vi "2P_AdapUprite_Linlin.vi"() -> ()   [LabVIEW 2015] (continued)
                                }
                                }
                                }
                                n1665 = Build Array(w4642) -> (w4641:T20)
                                }
                                }
                                }
                                frame #9 {
                                n1666 = Build Array(w4671, w4670) -> (w4673:bool[])
                                n1667 = Boolean Array To Number(Boolean array=w4673) -> (number=w4672:u32)
                                n1668 = case shown="0" w4672 {
                                tunnel: w4669 -> [_ w4725 _ w4729]
                                tunnel: [_ w4720 _ w4726] -> w4668
                                frame 1 {
                                n1669 = call "2pparameters.vi"("command"="get") -> ("params out"=w4680:T12)  [unwired: 1 in]
                                n1670 = Unbundle By Name(w4680) -> ("wavdet"=w4681:bool, "Pel"=w4683:sgl, "refwfsize"=w4684:dbl, "Pel"=w4682:sgl)
                                n1671 = call "waveformsDObuffer.vi"("command"="get") -> ("DO wf out"=w4676:digitalwaveform[])  [unwired: 1 in]
                                n1672 = case shown="True" w4681 {
                                tunnel: [w4688 w4701] -> w4678
                                tunnel: w4682 -> [w4697 w4716]
                                tunnel: w4683 -> [w4687 w4707]
                                tunnel: w4684 -> [_ w4713]
                                frame False {
                                w4691 = u16 0 items=["unsigned binary", "offset binary", "2's complement"] ("data format (offset binary)")
                                n1673 = Initialize Array(sgl 0.0, w4687) -> (w4694:sgl[])
                                n1674 = Replace Array Subset(array=w4694, new element=sgl 1.0, index=0) -> (w4692:sgl[])
                                n1675 = Reciprocal(x=w4697) -> (1/x=w4698:sgl)
                                n1676 = Bundle By Name("Y"=w4692, "dt"=w4698) -> (w4689:waveform(sgl))  [unwired: 1 in]
                                n1677 = call-poly <vilib>:"Analog to Digital.vi"("data format (offset binary)"=w4691, "compress digital (T)"=TRUE, "full-scale range (pk-pk)"=1.0, "resolution (16 bit)"=1, "analog waveform"=w4689) -> ("digital waveform"=w4688:digitalwaveform)  [unwired: 3 in, 3 out]
                                }
                                frame True {
                                w4704 = u16 0 items=["unsigned binary", "offset binary", "2's complement"] ("data format (offset binary)")
                                n1678 = To Double Precision Float(number=w4707) -> (double precision float=w4714:dbl)
                                n1679 = Initialize Array(sgl 0.0, w4707) -> (w4709:sgl[])
                                n1680 = Divide(x=w4713, y=w4714) -> (x/y=w4711:dbl)
                                n1681 = Round Toward +Infinity(x=w4711) -> (ceil(x): smallest int >= x=w4712:dbl)
                                n1682 = Replace Array Subset(array=w4709, new element=sgl 1.0, index=0) -> (w4706:sgl[])
                                n1683 = for {
                                N: w4712 -> [_]
                                tunnel: w4706 -> [w4718]
                                tunnel: [w4718] -> w4715 mode=concatenating
                                }
                                n1684 = Reciprocal(x=w4716) -> (1/x=w4717:sgl)
                                n1685 = Bundle By Name("Y"=w4715, "dt"=w4717) -> (w4702:waveform(sgl))  [unwired: 1 in]
                                n1686 = call-poly <vilib>:"Analog to Digital.vi"("data format (offset binary)"=w4704, "compress digital (T)"=TRUE, "full-scale range (pk-pk)"=1.0, "resolution (16 bit)"=1, "analog waveform"=w4702) -> ("digital waveform"=w4701:digitalwaveform)  [unwired: 3 in, 3 out]
                                }
                                }
                                n1687 = Build Array (concatenate)(w4676, w4678) -> (w4674:digitalwaveform[])
                                n1688 = call "waveformsDObuffer.vi"("DO wf in"=w4674, "command"="set") -> ()  [unwired: 1 out]
                                }
                                frame 2 {
                                n1689 = call "waveformsDObuffer.vi"("command"="get") -> ("DO wf out"=w4722:digitalwaveform[])  [unwired: 1 in]
                                n1690 = Delete From Array(array=w4722, length=1, index=w4725) -> (deleted portion=w4720:digitalwaveform[], array with subset deleted=w4719:digitalwaveform[])
                                n1691 = call "waveformsDObuffer.vi"("DO wf in"=w4719, "command"="set") -> ()  [unwired: 1 out]
                                }
                                frame 3, Default {
                                }
                                frame 0 {
                                n1692 = local read "Measurement"() -> (w4728:T4)
                                n1693 = To Unsigned Long Integer(number=w4728) -> (unsigned 32bit integer=w4727:u32)
                                n1694 = case shown="5..7" w4727 {
                                tunnel: w4729 -> [_ w4732]
                                tunnel: [_ w4731] -> w4726
                                frame 0..4, Default {
                                }
                                frame 5..7 {
                                n1695 = call "2pparameters.vi"("command"="get") -> ("params out"=w4739:T12)  [unwired: 1 in]
                                n1696 = Unbundle By Name(w4739) -> ("wavdet"=w4740:bool, "Pel"=w4742:sgl, "refwfsize"=w4743:dbl, "srateAODO"=w4741:sgl)
                                n1697 = call "waveformsDObuffer.vi"("command"="get") -> ("DO wf out"=w4733:digitalwaveform[])  [unwired: 1 in]
                                n1698 = Index Array(array=w4733, index=w4732) -> (element=w4734:digitalwaveform)
                                n1699 = case shown="True" w4740 {
                                tunnel: [w4747 w4760] -> w4737
                                tunnel: w4741 -> [w4756 w4775]
                                tunnel: w4742 -> [w4746 w4766]
                                tunnel: w4743 -> [_ w4772]
                                frame False {
                                w4750 = u16 0 items=["unsigned binary", "offset binary", "2's complement"] ("data format (offset binary)")
                                n1700 = Initialize Array(sgl 0.0, w4746) -> (w4753:sgl[])
                                n1701 = Replace Array Subset(array=w4753, new element=sgl 1.0, index=0) -> (w4751:sgl[])
                                n1702 = Reciprocal(x=w4756) -> (1/x=w4757:sgl)
                                n1703 = Bundle By Name("Y"=w4751, "dt"=w4757) -> (w4748:waveform(sgl))  [unwired: 1 in]
                                n1704 = call-poly <vilib>:"Analog to Digital.vi"("data format (offset binary)"=w4750, "compress digital (T)"=TRUE, "full-scale range (pk-pk)"=1.0, "resolution (16 bit)"=1, "analog waveform"=w4748) -> ("digital waveform"=w4747:digitalwaveform)  [unwired: 3 in, 3 out]
                                }
                                frame True {
                                w4763 = u16 0 items=["unsigned binary", "offset binary", "2's complement"] ("data format (offset binary)")
                                n1705 = To Double Precision Float(number=w4766) -> (double precision float=w4773:dbl)
                                n1706 = Initialize Array(sgl 0.0, w4766) -> (w4768:sgl[])
                                n1707 = Divide(x=w4772, y=w4773) -> (x/y=w4770:dbl)
                                n1708 = Round Toward +Infinity(x=w4770) -> (ceil(x): smallest int >= x=w4771:dbl)
                                n1709 = Replace Array Subset(array=w4768, new element=sgl 1.0, index=0) -> (w4765:sgl[])
                                n1710 = for {
                                N: w4771 -> [_]
                                tunnel: w4765 -> [w4777]
                                tunnel: [w4777] -> w4774 mode=concatenating
                                }
                                n1711 = Reciprocal(x=w4775) -> (1/x=w4776:sgl)
                                n1712 = Bundle By Name("Y"=w4774, "dt"=w4776) -> (w4761:waveform(sgl))  [unwired: 1 in]
                                n1713 = call-poly <vilib>:"Analog to Digital.vi"("data format (offset binary)"=w4763, "compress digital (T)"=TRUE, "full-scale range (pk-pk)"=1.0, "resolution (16 bit)"=1, "analog waveform"=w4761) -> ("digital waveform"=w4760:digitalwaveform)  [unwired: 3 in, 3 out]
                                }
                                }
                                n1714 = Build Array(w4734) -> (w4731:digitalwaveform[])
                                n1715 = Replace Array Subset(array=w4733, new element=w4737, index=w4732) -> (w4730:digitalwaveform[])
                                n1716 = call "waveformsDObuffer.vi"("DO wf in"=w4730, "command"="set") -> ()  [unwired: 1 out]
                                }
                                }
                                }
                                }
                                }
                                frame #10 {
                                # "Source of crashing?"
                                n1717 = local read "Meastab"() -> (w4791:enum32{"X-Y Image", "Linescan", "Timetrace"})
                                n1718 = property on="refwf" class="Ring (strict)"() -> ("RingText.Text"=w4788:string)  [unwired: 2 in, 2 out]
                                n1719 = case shown="\"Timetrace\"" w4791 {
                                tunnel: [w4793 w4794] -> w4792
                                frame "X-Y Image", Default {
                                n1720 = local read "Sampling rate"() -> (w4793:dbl)
                                }
                                frame "Timetrace" {
                                n1721 = local read "srateAODOtt"() -> (w4794:dbl)
                                }
                                }
                                n1722 = call "waveformsAObuffer.vi"("command"="get") -> ("AO wf out"=w4781:waveform(dbl)[])  [unwired: 1 in]
                                n1723 = local read "wavdet"() -> (w4789:bool)
                                n1724 = call "waveformsDObuffer.vi"("command"="get") -> ("DO wf out"=w4785:digitalwaveform[])  [unwired: 1 in]
                                n1725 = call "correctwaveformsizetemp.vi"("new sampling frequency (Hz)"=w4792, "start"=TRUE, "reference waveforms to"=w4788, "Analog waveforms in"=w4781, "stop"=FALSE, "Digital waveforms in"=w4785) -> ("analog wf out"=w4787:waveform(dbl)[], "Digital wf out"=w4780:digitalwaveform[], "measpoints"=w4790:i32)
                                n1726 = call "waveformsDObuffer.vi"("DO wf in"=w4780, "command"="set") -> ()  [unwired: 1 out]
                                n1727 = call "waveformsAObuffer.vi"("AO wf in"=w4787, "command"="set") -> ()  [unwired: 1 out]
                                n1728 = case shown="True" w4789 {
                                tunnel: w4790 -> [_ w4797]
                                tunnel: w4780 -> [_ w4795]
                                frame False {
                                }
                                frame True {
                                n1729 = local write "# of frames"(w4797) -> ()
                                n1730 = call "GetNumCamFramesv2.vi"("Digital Waveform Graph"=w4795) -> ("Numeric"=w4796:i32)  [unwired: 10 in]
                                n1731 = local write "Total Camera Frames"(w4796) -> ()
                                }
                                }
                                }
                                }
                              }
                              frame #7 {
                                # "Disabled for conversion to 64 bit"
                                # "lifetime related stuff"
                                n1732 = disable-structure shown="Disabled" {
                                frame Disabled {
                                n1733 = local read "Measurement"() -> (w4799:T4)
                                n1734 = case shown="\"Lifetime (scan)\"" w4799 {
                                frame "X-Y-t movie", Default {
                                }
                                frame "Lifetime (scan)" {
                                # "total acquisition time"
                                n1735 = call "2pparameters.vi"("command"="get") -> ("params out"=w4807:T12)  [unwired: 1 in]
                                n1736 = Unbundle By Name(w4807) -> ("measpoints"=w4801:i32, "srateAODO"=w4822:sgl)
                                n1737 = Divide(x=w4801, y=w4822) -> (x/y=w4800:sgl)
                                n1738 = local read "min phot"() -> (w4817:u32)
                                n1739 = local read "expected c/s"() -> (w4818:dbl)
                                n1740 = Multiply(x=w4800, y=1000.0) -> (x*y=w4810:dbl)
                                n1741 = local read "truncate"() -> (w4816:u32)
                                n1742 = To Long Integer(number=w4810) -> (32bit integer=w4819:i32)
                                n1743 = To Long Integer(number=w4818) -> (32bit integer=w4820:i32)
                                n1744 = local read "Number of Bins"() -> (w4811:u32)
                                n1745 = local read item#-1() -> (w4815)
                                n1746 = local write "Acquisition time"(w4819) -> ()
                                n1747 = local read item#-1() -> (w4813)
                                n1748 = local read item#-1() -> (w4814)
                                n1749 = local read item#-1() -> (w4812)
                                n1750 = call "lifetimeparameters.vi"("command"="get") -> ("Params out"=w4805:T22)  [unwired: 1 in]
                                n1751 = Add(x=100, y=w4819) -> (x+y=w4809:i32)
                                n1752 = Bundle By Name(cluster=w4805, "acq time"=w4809, "acq rate"=w4820, "# bins"=w4811, "Ch0 Level"=w4812, "Ch1 Level"=w4813, "Ch0 ZeroX"=w4814, "Ch1 ZeroX"=w4815, "min photons"=w4817, "truncate"=w4816) -> (w4804:T22)
                                n1753 = local write "Acquisition rate"(w4820) -> ()
                                n1754 = call "lifetimeparameters.vi"("Params in"=w4804, "command"="set") -> ()  [unwired: 1 out]
                                }
                                }
                                }
                                frame Enabled {
                                }
                                }
                                n1755 = local write "64bit disabled"(TRUE ("64bit disabled")) -> ()
                              }
                              frame #8 {
                                # "setting timeout and sample mode"
                                n1756 = call "2pparameters.vi"("command"="get") -> ("params out"=w4833:T12)  [unwired: 1 in]
                                n1757 = Unbundle By Name(w4833) -> ("refreshbuffer"=w4831:i32, "srate"=w4832:sgl)
                                n1758 = local read "wavdet"() -> (w4823:bool)
                                n1759 = To Double Precision Float(number=w4832) -> (double precision float=w4835:dbl)
                                n1760 = To Double Precision Float(number=w4831) -> (double precision float=w4826:dbl)
                                n1761 = case shown="False" w4823 {
                                tunnel: [w4840 w4841] -> w4825
                                frame False {
                                w4840 = 10123 items=["Finite Samples"=10178, "Continuous Samples"=10123, "Hardware Timed Single Point"=12522] ("sample mode")
                                }
                                frame True {
                                w4841 = 10123 items=["Finite Samples"=10178, "Continuous Samples"=10123, "Hardware Timed Single Point"=12522] ("sample mode")
                                }
                                }
                                n1762 = Divide(x=w4826, y=w4835) -> (x/y=w4839:dbl)
                                n1763 = Multiply(x=w4839, y=2.0) -> (x*y=w4836:dbl)
                                n1764 = Max & Min(x=w4836, y=10.0) -> (max(x,y)=w4827:dbl)  [unwired: 1 out]
                                n1765 = call "2pparameters.vi"("command"="get") -> ("params out"=w4830:T12)  [unwired: 1 in]
                                n1766 = Bundle By Name(cluster=w4830, "timeout"=w4827, "sample mode"=w4825) -> (w4828:T12)
                                n1767 = call "2pparameters.vi"("Params in"=w4828, "command"="set") -> ()  [unwired: 1 out]
                              }
                            }
                          }
                          frame #1 {
                            # "waveform prepped in prep AO img"
                            # "Disabled for conversion to 64 bit"
                            # "start preparing the tasks"
                            n1768 = call "prepAO_img.vi"() -> ("Terminal Name with Device Prefix"=w4843:tag)
                            n1769 = call "prepDO_img.vi"() -> ()  [unwired: 2 in]
                            n1770 = call "prepAI_img.vi"("triggersource"=w4843) -> ()  [unwired: 2 in]
                            n1771 = call "prepCI_img.vi"("ArmStart.DigEdge.Src"=w4843) -> ()  [unwired: 1 in]
                            n1772 = disable-structure shown="Disabled" {
                              frame Disabled {
                                n1773 = local read "Measurement"() -> (w4844:T4)
                                n1774 = case shown="\"Lifetime (contour)\"" w4844 {
                                frame "X-Y-t movie", Default {
                                }
                                frame "Lifetime (contour)" {
                                n1775 = stacked-sequence {
                                frame #0 {
                                n1776 = call "PH-temp.vi"("String"="clear" ("command")) -> ()  [unwired: 2 in, 2 out]
                                n1777 = call "PH-temp-raw.vi"("command"="empty") -> ()  [unwired: 1 in, 1 out]
                                }
                                frame #1 {
                                n1778 = call "calib.vi"() -> ()  [unwired: 1 in]
                                }
                                frame #2 {
                                n1779 = call "setup.vi"() -> ()  [unwired: 1 in]
                                }
                                }
                                }
                                }
                              }
                              frame Enabled {
                              }
                            }
                            n1780 = local write "64bit disabled"(TRUE ("64bit disabled")) -> ()
                          }
                          frame #2 {
                            # "prepares files for saving"
                            n1781 = local read "save\ndata"() -> (w4847:bool)
                            n1782 = case shown="True" w4847 {
                              tunnel: w4848 -> [_ w4852]
                              frame False {
                              }
                              frame True {
                                n1783 = local read "filename prefix"() -> (w4850:string)
                                n1784 = local read "data dir"() -> (w4851:path)
                                n1785 = call "preparebinaryfiles.vi"("filename prefix"=w4850, "data dir"=w4851, "timestamp"=w4852) -> ("full-filename"=w4849:string)  [unwired: 1 in]
                                n1786 = local write "full-filename"(w4849) -> ()
                              }
                            }
                            n1787 = call "preptempbuffers_tt.vi"() -> ()  [unwired: 12 in]
                          }
                          frame #3 {
                            n1788 = local read "wavdet"() -> (w4853:bool)
                            n1789 = case shown="False" w4853 {
                              frame False {
                                n1790 = disable-structure shown="Disabled" {
                                frame Disabled {
                                n1791 = call "2pparameters.vi"("command"="get") -> ("params out"=w4856:T12)  [unwired: 1 in]
                                n1792 = Unbundle By Name(w4856) -> ("autoshutter"=w4857:bool, "aAS"=w4854:u32[])
                                n1793 = case shown="True" w4857 {
                                tunnel: w4854 -> [_ w4858]
                                frame False {
                                }
                                frame True {
                                n1794 = call "shuttercontrol_multi.vi"("Autoshutter Chans"=w4858, "command"="open") -> ()  [unwired: 1 in, 1 out]
                                }
                                }
                                }
                                frame Enabled {
                                }
                                }
                              }
                              frame True {
                              }
                            }
                          }
                          frame #4 {
                            # "start trigger comes from AO, so  start everything and then start AO"
                            n1795 = flat-sequence {
                              frame #0 {
                                # "Disabled for conversion to 64 bit"
                                n1796 = disable-structure shown="Disabled" {
                                frame Disabled {
                                n1797 = local read "Measurement"() -> (w4861:T4)
                                n1798 = case shown="\"Lifetime (contour)\"" w4861 {
                                frame "X-Y-t movie", Default {
                                }
                                frame "Lifetime (contour)" {
                                n1799 = call "runLT_img.vi"() -> ()  [unwired: 1 in]
                                }
                                }
                                }
                                frame Enabled {
                                }
                                }
                                n1800 = local write "64bit disabled"(TRUE ("64bit disabled")) -> ()
                              }
                              frame #1 {
                                n1801 = call "runAI_img.vi"() -> ()  [unwired: 12 in]
                                n1802 = call "runCI.vi"() -> ()  [unwired: 12 in]
                                n1803 = call "runDO_img.vi"() -> ()  [unwired: 12 in]
                              }
                              frame #2 {
                                n1804 = call "runAO_img.vi"() -> ()  [unwired: 12 in]
                              }
                            }
                          }
                          frame #5 {
                            # "Disabled for conversion to 64 bit"
                            n1805 = while {
                              i -> [w4887]
                              stop <- w4885 stop-if-true
                              n1806 = local read "Stop"() -> (w4895:bool)
                              n1807 = local read "Exit"() -> (w4894:bool)
                              n1808 = Or(x=w4895, y=w4894) -> (x .or. y?=w4893:bool)
                              n1809 = case shown="False" w4893 {
                                frame False {
                                n1810 = stacked-sequence {
                                frame #0 {
                                n1811 = call "collectAI_tt_V2.vi"() -> ()  [unwired: 4 in]
                                n1812 = call "collectCI_tt.vi"() -> ("size(s)"=w4902:i32)  [unwired: 3 in]
                                n1813 = local write "scol"(w4902) -> ()
                                }
                                frame #1 {
                                n1814 = local read "Live"() -> (w4903:bool)
                                n1815 = case shown="True" w4903 {
                                frame False {
                                }
                                frame True {
                                n1816 = local read "graph1list"() -> (w4910:u16)
                                n1817 = local read "graph2list"() -> (w4909:u16)
                                n1818 = To Unsigned Word Integer(number=w4910) -> (unsigned 16bit integer=w4908:u16)
                                n1819 = To Unsigned Word Integer(number=w4909) -> (unsigned 16bit integer=w4907:u16)
                                n1820 = call "dattotrace.vi"("graph2list"=w4907, "Current Average"=sgl 1.0, "graph1list"=w4908) -> ("trace2array out"=w4905:sgl[], "trace1array out"=w4916:sgl[])
                                n1821 = local read "bin"() -> (w4917:dbl)
                                n1822 = script code="data=reshape(datain,[bin length(datain)./bin]);\ndataout=mean(data,1);\ndata2=reshape(datain2,[bin length(datain2)./bin]);\ndataout2=mean(data2,1);"("bin"=w4917, "datain"=w4916, "datain2"=w4905) -> ("dataout"=w4915:dbl[], "dataout2"=w4904:dbl[])  [unwired: 1 in, 1 out]
                                n1823 = Array Size(array=w4904) -> (size(s)=w4918:i32)
                                n1824 = Divide(x=w4918, y=2) -> (x/y=w4920:dbl)
                                n1825 = Round To Nearest(number=w4920) -> (nearest integer value=w4922:dbl)
                                n1826 = Array Size(array=w4915) -> (size(s)=w4927:i32)
                                n1827 = Delete From Array(array=w4904, length=w4922, index=0) -> (deleted portion=w4913:dbl[], array with subset deleted=w4914:dbl[])
                                n1828 = Divide(x=w4927, y=2) -> (x/y=w4925:dbl)
                                n1829 = Round To Nearest(number=w4925) -> (nearest integer value=w4923:dbl)
                                n1830 = Delete From Array(array=w4915, length=w4923, index=0) -> (deleted portion=w4912:dbl[], array with subset deleted=w4911:dbl[])
                                n1831 = local write "graph2"(w4911) -> ()
                                n1832 = local write "graph1"(w4912) -> ()
                                n1833 = local write "graph3"(w4913) -> ()
                                n1834 = local write "graph4"(w4914) -> ()
                                }
                                }
                                }
                                frame #2 {
                                n1835 = local read "save\ndata"() -> (w4928:bool)
                                n1836 = case shown="True" w4928 {
                                frame False {
                                }
                                frame True {
                                n1837 = call "savebinaryfiles.vi"() -> ()  [unwired: 1 in]
                                }
                                }
                                }
                                }
                                }
                                frame True {
                                }
                              }
                              n1838 = Increment(x=w4887) -> (x+1=w4886:i32)
                              n1839 = local write "points recorded"(w4886) -> ()
                              n1840 = local read "continuous"() -> (w4890:bool)
                              n1841 = case shown="False" w4890 {
                                tunnel: w4886 -> [w4900 _]
                                tunnel: [w4899 FALSE] -> w4888
                                frame False {
                                n1842 = call "2pparameters.vi"("command"="get") -> ("params out"=w4897:T12)  [unwired: 1 in]
                                n1843 = Unbundle By Name(w4897) -> ("tt_cycles"=w4896:i32)
                                n1844 = Greater Or Equal?(x=w4900, y=w4896) -> (x >= y?=w4899:bool)
                                }
                                frame True {
                                }
                              }
                              n1845 = local read "Stop"() -> (w4892:bool)
                              n1846 = local read "Exit"() -> (w4891:bool)
                              n1847 = Or(x=w4892, y=w4891) -> (x .or. y?=w4889:bool)
                              n1848 = Or(x=w4889, y=w4888) -> (x .or. y?=w4885:bool)
                            }
                            n1849 = disable-structure shown="Disabled" {
                              disable-tunnel: w4863 -> [w4864 _]
                              frame Disabled {
                                w4867 = u16 0 items=["Stream to disk", "Post process", "real time process"] ("Ring")
                                n1850 = local read "T3R Data processing"() -> (w4866:u16)
                                n1851 = Equal?(x=w4866, y=w4867) -> (x = y?=w4865:bool)
                                n1852 = local read "save\ndata"() -> (w4869:bool)
                                n1853 = local read "Measurement"() -> (w4870:T4)
                                n1854 = And(x=w4869, y=w4865) -> (x .and. y?=w4868:bool)
                                n1855 = case shown="\"Lifetime (contour)\"" w4870 {
                                tunnel: w4864 -> [_ w4874]
                                tunnel: w4868 -> [_ w4872]
                                frame "X-Y-t movie", Default {
                                }
                                frame "Lifetime (contour)" {
                                n1856 = case shown="True" w4872 {
                                selector: w4872 -> [w4875 w4880]
                                tunnel: w4874 -> [_ w4878]
                                tunnel: [path "" ("appended path") w4881] -> w4873
                                tunnel: [w4875 w4880] -> w4871
                                frame False {
                                }
                                frame True {
                                n1857 = local read "filename prefix"() -> (w4879:string)
                                n1858 = local read "data dir"() -> (w4882:path)
                                n1859 = call "generatedatafilename.vi"("timestamp"=w4878, "filename prefix in"=w4879) -> ("full-filename"=w4877:string)
                                n1860 = Concatenate Strings(w4877, ".lvpt3contour" ("string")) -> (w4884:string)
                                n1861 = Build Path(base path=w4882, name or relative path=w4884) -> (appended path=w4881:path)
                                }
                                }
                                n1862 = call "collectLT_res_v1.vi"("stream?"=w4871, "data file"=w4873) -> ()  [unwired: 2 out]
                                }
                                }
                              }
                              frame Enabled {
                              }
                            }
                            n1863 = local write "64bit disabled"(TRUE ("64bit disabled")) -> ()
                          }
                          frame #6 {
                            # "Disabled for conversion to 64 bit"
                            n1864 = local read "Measurement"() -> (w4931:T4)
                            n1865 = disable-structure shown="Disabled" {
                              disable-tunnel: w4931 -> [w4933 _]
                              disable-tunnel: w4930 -> [w4932 _]
                              frame Disabled {
                                n1866 = case shown="\"Lifetime (contour)\"" w4933 {
                                tunnel: w4932 -> [_ w4934]
                                frame "X-Y-t movie", Default {
                                }
                                frame "Lifetime (contour)" {
                                n1867 = stacked-sequence {
                                tunnel: w4934 -> [_ w4935]
                                frame #0 {
                                n1868 = flat-sequence {
                                frame #0 {
                                n1869 = call "stoperaseLT_img.vi"() -> ()  [unwired: 1 in]
                                }
                                }
                                }
                                frame #1 {
                                w4938 = u16 0 items=["Stream to disk", "Post process", "real time process"] ("Ring")
                                n1870 = local read "T3R Data processing"() -> (w4937:u16)
                                n1871 = local read "save\ndata"() -> (w4940:bool)
                                n1872 = Equal?(x=w4937, y=w4938) -> (x = y?=w4936:bool)
                                n1873 = Not(x=w4936) -> (.not. x?=w4941:bool)
                                n1874 = And(x=w4940, y=w4941) -> (x .and. y?=w4939:bool)
                                n1875 = case shown="True" w4939 {
                                tunnel: w4935 -> [_ w4942]
                                frame False {
                                }
                                frame True {
                                n1876 = local read "filename prefix"() -> (w4943:string)
                                n1877 = local read "data dir"() -> (w4959:path)
                                n1878 = call "2pparameters.vi"("command"="get") -> ("params out"=w4954:T12)  [unwired: 1 in]
                                n1879 = call "generatedatafilename.vi"("timestamp"=w4942, "filename prefix in"=w4943) -> ("full-filename"=w4944:string)
                                n1880 = Unbundle By Name(w4954) -> ("srate"=w4952:sgl, "Pel"=w4951:sgl, "measpoints"=w4949:i32)
                                n1881 = Concatenate Strings(w4944, ".lvpt3contour" ("string")) -> (w4957:string)
                                n1882 = Build Path(base path=w4959, name or relative path=w4957) -> (appended path=w4956:path)
                                n1883 = To Unsigned Long Integer(number=w4952) -> (unsigned 32bit integer=w4953:u32)
                                n1884 = To Unsigned Long Integer(number=w4951) -> (unsigned 32bit integer=w4950:u32)
                                n1885 = To Unsigned Long Integer(number=w4949) -> (unsigned 32bit integer=w4948:u32)
                                n1886 = call "PH-temp-raw.vi"("command"="get") -> ("array out"=w4947:u32[])  [unwired: 1 in]
                                n1887 = Build Array (concatenate)(w4953, w4950, w4948, w4947) -> (w4946:u32[])
                                n1888 = Open/Create/Replace File(file path (use dialog)=w4956, operation (0:open)=T9."replace or create") -> (refnum out=w4963:refnum<file>, error out=w4962:errorcluster)  [unwired: 4 in, 1 out]
                                n1889 = Write to Binary File(file (use dialog)=w4963, data=w4946, error in=w4962, 5:FALSE ("prepend array or string size? (T)")) -> (refnum out=w4960:refnum<file>, error out=w4961:errorcluster)  [unwired: 2 in, 1 out]
                                n1890 = Close File(refnum=w4960, error in=w4961) -> ()  [unwired: 2 out]
                                }
                                }
                                }
                                }
                                }
                                }
                              }
                              frame Enabled {
                              }
                            }
                            n1891 = local write "64bit disabled"(TRUE ("64bit disabled")) -> ()
                          }
                          frame #7 {
                            n1892 = flat-sequence {
                              frame #0 {
                                n1893 = call "reset AO_DO_v3.vi"() -> ()  [unwired: 12 in]
                              }
                              frame #1 {
                                n1894 = call "stoperaseCI.vi"() -> ()  [unwired: 12 in]
                                n1895 = call "stoperaseDO_img.vi"() -> ()  [unwired: 12 in]
                                n1896 = call "stoperaseAO_img.vi"() -> ()  [unwired: 12 in]
                                n1897 = call "stoperaseAI_img.vi"() -> ()  [unwired: 12 in]
                              }
                            }
                          }
                          frame #8 {
                            n1898 = stacked-sequence {
                              tunnel: w4979 -> [w4982 _ _ _ _ _]
                              tunnel: w4976 -> [w4981 _ _ _ _ _]
                              tunnel: w4977 -> [w4980 _ _ _ _ _]
                              tunnel: w4978 -> [_ w5031 _ _ _ _]
                              tunnel: w4974 -> [_ w5030 w5081 w5202 _ _]
                              tunnel: w4975 -> [_ w5029 w5082 w5201 _ _]
                              tunnel: w4973 -> [_ _ _ w5200 _ _]
                              tunnel: w4972 -> [_ _ _ w5199 _ _]
                              tunnel: w4971 -> [_ _ w5084 _ _ _]
                              tunnel: w4970 -> [_ _ w5083 _ _ _]
                              tunnel: w4969 -> [_ _ w5078 _ _ _]
                              tunnel: w4968 -> [_ _ w5079 _ _ _]
                              tunnel: w4967 -> [_ _ _ w5197 _ _]
                              tunnel: w4966 -> [_ _ _ w5196 _ _]
                              frame #0 {
                                n1899 = case shown="False" w4982 {
                                tunnel: w4981 -> [_ w5004]
                                tunnel: w4980 -> [_ w5003]
                                frame True {
                                n1900 = stacked-sequence {
                                seq-local: [w4985 _ _] -> [_ w4995 w5000]
                                frame #0 {
                                n1901 = call "configuration_2P_Linlin.vi"("command"="get") -> ("config out"=w4984:T14)  [unwired: 2 in, 1 out]
                                n1902 = Unbundle By Name(w4984) -> ("Voltage to Xgalvo"=w4988:i32)
                                n1903 = call "2pparameters.vi"("command"="get") -> ("params out"=w4989:T12)  [unwired: 1 in]
                                n1904 = in-place {
                                in-place-border: w4988 -> [w4994]
                                in-place-border: [w4991] -> w4985
                                n1905 = in-place-cluster #31(w4989) -> ("aAO"=w4993:u32[])
                                n1906 = call "remove channel from active arrayv2.vi"("line array in"=w4993, "line to remove"=w4994) -> ("line array out"=w4992:u32[], "index"=w4991:i32)  [unwired: 1 out]
                                n1907 = in-place-cluster #31("aAO"=w4992) -> (w4986:T12)
                                }
                                n1908 = call "2pparameters.vi"("Params in"=w4986, "command"="set") -> ()  [unwired: 1 out]
                                }
                                frame #1 {
                                n1909 = call "waveformparamsv2.vi"("command"="rem AO", "index"=w4995) -> ()  [unwired: 3 in, 3 out]
                                }
                                frame #2 {
                                n1910 = call "waveformsAObuffer.vi"("command"="get") -> ("AO wf out"=w5001:waveform(dbl)[])  [unwired: 1 in]
                                n1911 = Delete From Array(array=w5001, length=1, index=w5000) -> (array with subset deleted=w4997:waveform(dbl)[])  [unwired: 1 out]
                                n1912 = call "waveformsAObuffer.vi"("AO wf in"=w4997, "command"="set") -> ()  [unwired: 1 out]
                                }
                                }
                                }
                                frame False {
                                n1913 = stacked-sequence {
                                seq-local: [w5007 _ _] -> [_ w5013 w5024]
                                tunnel: w5004 -> [_ w5012 _]
                                tunnel: w5003 -> [_ _ w5023]
                                frame #0 {
                                n1914 = call "configuration_2P_Linlin.vi"("command"="get") -> ("config out"=w5005:T14)  [unwired: 2 in, 1 out]
                                n1915 = Unbundle By Name(w5005) -> ("Voltage to Xgalvo"=w5008:i32)
                                n1916 = call "2pparameters.vi"("command"="get") -> ("params out"=w5011:T12)  [unwired: 1 in]
                                n1917 = Unbundle By Name(w5011) -> ("aAO"=w5009:u32[])
                                n1918 = Search 1D Array(1D array=w5009, element=w5008) -> (index of element=w5007:i32)  [unwired: 1 in]
                                }
                                frame #1 {
                                n1919 = call "waveformparamsv2.vi"("command"="get") -> ("Params out"=w5016:T17)  [unwired: 4 in, 2 out]
                                n1920 = in-place {
                                in-place-border: w5013 -> [w5020]
                                in-place-border: w5012 -> [w5019]
                                n1921 = in-place-cluster #32(w5016) -> ("AO parameters"=w5021:T18)
                                n1922 = in-place {
                                in-place-border: w5019 -> [w5022]
                                n1923 = in-place-array #33(w5021, w5020) -> ()  [unwired: 1 out]
                                n1924 = in-place-array #33(w5022) -> (w5018:T18)  [unwired: 1 out]
                                }
                                n1925 = in-place-cluster #32("AO parameters"=w5018) -> (w5014:T17)
                                }
                                n1926 = call "waveformparamsv2.vi"("command"="set", "Params in"=w5014) -> ()  [unwired: 3 in, 3 out]
                                }
                                frame #2 {
                                n1927 = call "waveformsAObuffer.vi"("command"="get") -> ("AO wf out"=w5027:waveform(dbl)[])  [unwired: 1 in]
                                n1928 = Replace Array Subset(array=w5027, new element=w5023, index=w5024) -> (w5025:waveform(dbl)[])
                                n1929 = call "waveformsAObuffer.vi"("AO wf in"=w5025, "command"="set") -> ()  [unwired: 1 out]
                                }
                                }
                                }
                                }
                              }
                              frame #1 {
                                n1930 = case shown="False" w5031 {
                                tunnel: w5030 -> [_ w5053]
                                tunnel: w5029 -> [_ w5052]
                                frame True {
                                n1931 = stacked-sequence {
                                seq-local: [w5034 _ _] -> [_ w5044 w5049]
                                frame #0 {
                                n1932 = call "configuration_2P_Linlin.vi"("command"="get") -> ("config out"=w5032:T14)  [unwired: 2 in, 1 out]
                                n1933 = Unbundle By Name(w5032) -> ("Voltage to Ygalvo"=w5037:i32)
                                n1934 = call "2pparameters.vi"("command"="get") -> ("params out"=w5038:T12)  [unwired: 1 in]
                                n1935 = in-place {
                                in-place-border: w5037 -> [w5043]
                                in-place-border: [w5040] -> w5034
                                n1936 = in-place-cluster #34(w5038) -> ("aAO"=w5042:u32[])
                                n1937 = call "remove channel from active arrayv2.vi"("line array in"=w5042, "line to remove"=w5043) -> ("line array out"=w5041:u32[], "index"=w5040:i32)  [unwired: 1 out]
                                n1938 = in-place-cluster #34("aAO"=w5041) -> (w5035:T12)
                                }
                                n1939 = call "2pparameters.vi"("Params in"=w5035, "command"="set") -> ()  [unwired: 1 out]
                                }
                                frame #1 {
                                n1940 = call "waveformparamsv2.vi"("command"="rem AO", "index"=w5044) -> ()  [unwired: 3 in, 3 out]
                                }
                                frame #2 {
                                n1941 = call "waveformsAObuffer.vi"("command"="get") -> ("AO wf out"=w5050:waveform(dbl)[])  [unwired: 1 in]
                                n1942 = Delete From Array(array=w5050, length=1, index=w5049) -> (array with subset deleted=w5046:waveform(dbl)[])  [unwired: 1 out]
                                n1943 = call "waveformsAObuffer.vi"("AO wf in"=w5046, "command"="set") -> ()  [unwired: 1 out]
                                }
                                }
                                }
                                frame False {
                                n1944 = stacked-sequence {
                                seq-local: [w5056 _ _] -> [_ w5062 w5073]
                                tunnel: w5053 -> [_ w5061 _]
                                tunnel: w5052 -> [_ _ w5072]
                                frame #0 {
                                n1945 = call "configuration_2P_Linlin.vi"("command"="get") -> ("config out"=w5054:T14)  [unwired: 2 in, 1 out]
                                n1946 = Unbundle By Name(w5054) -> ("Voltage to Ygalvo"=w5057:i32)
                                n1947 = call "2pparameters.vi"("command"="get") -> ("params out"=w5060:T12)  [unwired: 1 in]
                                n1948 = Unbundle By Name(w5060) -> ("aAO"=w5058:u32[])
                                n1949 = Search 1D Array(1D array=w5058, element=w5057) -> (index of element=w5056:i32)  [unwired: 1 in]
                                }
                                frame #1 {
                                n1950 = call "waveformparamsv2.vi"("command"="get") -> ("Params out"=w5065:T17)  [unwired: 4 in, 2 out]
                                n1951 = in-place {
                                in-place-border: w5062 -> [w5069]
                                in-place-border: w5061 -> [w5068]
                                n1952 = in-place-cluster #35(w5065) -> ("AO parameters"=w5070:T18)
                                n1953 = in-place {
                                in-place-border: w5068 -> [w5071]
                                n1954 = in-place-array #36(w5070, w5069) -> ()  [unwired: 1 out]
                                n1955 = in-place-array #36(w5071) -> (w5067:T18)  [unwired: 1 out]
                                }
                                n1956 = in-place-cluster #35("AO parameters"=w5067) -> (w5063:T17)
                                }
                                n1957 = call "waveformparamsv2.vi"("command"="set", "Params in"=w5063) -> ()  [unwired: 3 in, 3 out]
                                }
                                frame #2 {
                                n1958 = call "waveformsAObuffer.vi"("command"="get") -> ("AO wf out"=w5076:waveform(dbl)[])  [unwired: 1 in]
                                n1959 = Replace Array Subset(array=w5076, new element=w5072, index=w5073) -> (w5074:waveform(dbl)[])
                                n1960 = call "waveformsAObuffer.vi"("AO wf in"=w5074, "command"="set") -> ()  [unwired: 1 out]
                                }
                                }
                                }
                                }
                              }
                              frame #2 {
                                n1961 = Build Array(w5084, w5083) -> (w5085:bool[])
                                n1962 = Boolean Array To Number(Boolean array=w5085) -> (number=w5080:u32)
                                n1963 = case shown="2" w5080 {
                                tunnel: w5081 -> [_ _ w5143]
                                tunnel: w5082 -> [_ _ w5142]
                                tunnel: w5078 -> [_ w5115 w5140]
                                tunnel: w5079 -> [_ w5114 w5141]
                                frame 1, Default {
                                n1964 = stacked-sequence {
                                seq-local: [w5088 _ _] -> [_ w5100 w5105]
                                frame #0 {
                                # "Remove autoshutter channel from DO list in 2p parameters"
                                n1965 = call "2pparameters.vi"("command"="get") -> ("params out"=w5087:T12)  [unwired: 1 in]
                                n1966 = Unbundle By Name(w5087) -> ("aAS"=w5086:u32[])
                                n1967 = for {
                                tunnel: [w5094] -> w5088 mode=indexing
                                tunnel: w5086 -> [w5092] mode=indexing
                                shift-right: [w5095] -> w5089
                                shift-left: w5087 -> [w5093]
                                n1968 = in-place {
                                in-place-border: w5092 -> [w5099]
                                in-place-border: [w5096] -> w5094
                                n1969 = in-place-cluster #37(w5093) -> ("aDO"=w5098:u32[])
                                n1970 = call "remove channel from active arrayv2.vi"("line array in"=w5098, "line to remove"=w5099) -> ("line array out"=w5097:u32[], "index"=w5096:i32)  [unwired: 1 out]
                                n1971 = in-place-cluster #37("aDO"=w5097) -> (w5095:T12)
                                }
                                }
                                n1972 = call "2pparameters.vi"("Params in"=w5089, "command"="set") -> ()  [unwired: 1 out]
                                }
                                frame #1 {
                                n1973 = for {
                                tunnel: w5100 -> [w5101] mode=indexing
                                n1974 = call "waveformparamsv2.vi"("command"="rem DO", "index"=w5101) -> ()  [unwired: 3 in, 3 out]
                                }
                                }
                                frame #2 {
                                # "sort so it removes the last elements first\nand does not mess up the order"
                                # "Remove waveforms of autoshutter channels from wave forms DO"
                                n1975 = call "waveformsDObuffer.vi"("command"="get") -> ("DO wf out"=w5108:digitalwaveform[])  [unwired: 1 in]
                                n1976 = Sort 1D Array(array=w5105) -> (sorted array=w5104:i32[])
                                n1977 = Reverse 1D Array(array=w5104) -> (reversed array=w5103:i32[])
                                n1978 = for {
                                tunnel: w5103 -> [w5110] mode=indexing
                                shift-right: [w5111] -> w5106
                                shift-left: w5108 -> [w5113]
                                n1979 = Delete From Array(array=w5113, length=1, index=w5110) -> (array with subset deleted=w5111:digitalwaveform[])  [unwired: 1 out]
                                }
                                n1980 = call "waveformsDObuffer.vi"("DO wf in"=w5106, "command"="set") -> ()  [unwired: 1 out]
                                }
                                }
                                }
                                frame 2 {
                                n1981 = stacked-sequence {
                                tunnel: w5115 -> [_ w5127 _]
                                tunnel: w5114 -> [_ _ w5134]
                                frame #0 {
                                # "add autoshutter channels to digital out"
                                n1982 = call "2pparameters.vi"("command"="get") -> ("params out"=w5117:T12)  [unwired: 1 in]
                                n1983 = Unbundle By Name(w5117) -> ("aAS"=w5116:u32[])
                                n1984 = in-place {
                                in-place-border: w5116 -> [w5121]
                                n1985 = in-place-cluster #38(w5117) -> ("aDO"=w5123:u32[])
                                n1986 = for {
                                shift-right: [w5125] -> w5122
                                shift-left: w5123 -> [w5126]
                                tunnel: w5121 -> [w5124] mode=indexing
                                n1987 = call "add channel to active arrayv2.vi"("line array in"=w5126, "line to add"=w5124) -> ("line array out"=w5125:u32[])  [unwired: 2 out]
                                }
                                n1988 = in-place-cluster #38("aDO"=w5122) -> (w5118:T12)
                                }
                                n1989 = call "2pparameters.vi"("Params in"=w5118, "command"="set") -> ()  [unwired: 1 out]
                                }
                                frame #1 {
                                # "Not sure the correct way to add multiple sets of parameters..."
                                # "add autoshutter waveforms to wf parameters v2"
                                n1990 = disable-structure shown="Disabled" {
                                disable-tunnel: w5127 -> [w5129 _]
                                frame Disabled {
                                n1991 = for {
                                tunnel: w5129 -> [w5130] mode=indexing
                                n1992 = call "waveformparamsv2.vi"("command"="add DO", "add DO"=w5130) -> ()  [unwired: 3 in, 3 out]
                                }
                                }
                                frame Enabled {
                                }
                                }
                                n1993 = call "waveformparamsv2.vi"("command"="add DO", "add DO"=w5127) -> ()  [unwired: 3 in, 3 out]
                                }
                                frame #2 {
                                # "add autoshutter waveforms to wave forms DO"
                                n1994 = call "waveformsDObuffer.vi"("command"="get") -> ("DO wf out"=w5135:digitalwaveform[])  [unwired: 1 in]
                                n1995 = for {
                                tunnel: w5134 -> [w5138] mode=indexing
                                shift-right: [w5137] -> w5132
                                shift-left: w5135 -> [w5139]
                                n1996 = Build Array (concatenate)(w5139, w5138) -> (w5137:digitalwaveform[])
                                }
                                n1997 = call "waveformsDObuffer.vi"("DO wf in"=w5132, "command"="set") -> ()  [unwired: 1 out]
                                }
                                }
                                }
                                frame 0 {
                                n1998 = stacked-sequence {
                                seq-local: [w5145 _ _] -> [_ w5153 w5177]
                                tunnel: w5143 -> [_ _ _]
                                tunnel: w5142 -> [_ _ _]
                                tunnel: w5141 -> [_ _ w5176]
                                tunnel: w5140 -> [_ w5152 _]
                                frame #0 {
                                n1999 = call "2pparameters.vi"("command"="get") -> ("params out"=w5148:T12)  [unwired: 1 in]
                                n2000 = Unbundle By Name(w5148) -> ("aDO"=w5146:u32[], "aAS"=w5144:u32[])
                                n2001 = for {
                                tunnel: w5146 -> [w5151]
                                tunnel: [w5150] -> w5145 mode=indexing
                                tunnel: w5144 -> [w5149] mode=indexing
                                n2002 = Search 1D Array(1D array=w5151, element=w5149) -> (index of element=w5150:i32)  [unwired: 1 in]
                                }
                                }
                                frame #1 {
                                n2003 = call "2pparameters.vi"("command"="get") -> ("params out"=w5156:T12)  [unwired: 1 in]
                                n2004 = Unbundle By Name(w5156) -> ("wavdet"=w5154:bool, "autoshutter"=w5155:bool)
                                n2005 = case shown="True" w5155 {
                                tunnel: w5153 -> [_ w5160]
                                tunnel: w5154 -> [_ w5159]
                                tunnel: w5152 -> [_ w5158]
                                frame False {
                                }
                                frame True {
                                n2006 = case shown="False" w5159 {
                                tunnel: w5160 -> [w5162 _]
                                tunnel: w5158 -> [w5161 _]
                                frame False {
                                # "Replace autoshutter channel DO waveforms with those that were generated from autoshutter."
                                n2007 = call "waveformparamsv2.vi"("command"="get") -> ("Params out"=w5165:T17)  [unwired: 4 in, 2 out]
                                n2008 = in-place {
                                in-place-border: w5162 -> [w5169]
                                in-place-border: w5161 -> [w5167]
                                n2009 = in-place-cluster #39(w5165) -> ("DO parameters"=w5170:T20)
                                n2010 = for {
                                tunnel: w5169 -> [w5173] mode=indexing
                                tunnel: w5167 -> [w5171] mode=indexing
                                shift-right: [w5172] -> w5168
                                shift-left: w5170 -> [w5174]
                                n2011 = in-place {
                                in-place-border: w5171 -> [w5175]
                                n2012 = in-place-array #40(w5174, w5173) -> ()  [unwired: 1 out]
                                n2013 = in-place-array #40(w5175) -> (w5172:T20)  [unwired: 1 out]
                                }
                                }
                                n2014 = in-place-cluster #39("DO parameters"=w5168) -> (w5163:T17)
                                }
                                n2015 = call "waveformparamsv2.vi"("command"="set", "Params in"=w5163) -> ()  [unwired: 3 in, 3 out]
                                }
                                frame True {
                                }
                                }
                                }
                                }
                                }
                                frame #2 {
                                n2016 = call "2pparameters.vi"("command"="get") -> ("params out"=w5180:T12)  [unwired: 1 in]
                                n2017 = Unbundle By Name(w5180) -> ("wavdet"=w5178:bool, "autoshutter"=w5179:bool)
                                n2018 = case shown="True" w5179 {
                                tunnel: w5177 -> [_ w5184]
                                tunnel: w5178 -> [_ w5183]
                                tunnel: w5176 -> [_ w5182]
                                frame False {
                                }
                                frame True {
                                n2019 = case shown="False" w5183 {
                                tunnel: w5184 -> [w5186 _]
                                tunnel: w5182 -> [w5185 _]
                                frame False {
                                # "replace autoshutter channels of waveforms DO with autoshutter waveforms"
                                n2020 = call "waveformsDObuffer.vi"("command"="get") -> ("DO wf out"=w5188:digitalwaveform[])  [unwired: 1 in]
                                n2021 = for {
                                tunnel: w5186 -> [w5192] mode=indexing
                                tunnel: w5185 -> [w5191] mode=indexing
                                shift-right: [w5194] -> w5190
                                shift-left: w5188 -> [w5193]
                                n2022 = Replace Array Subset(array=w5193, new element=w5191, index=w5192) -> (w5194:digitalwaveform[])
                                }
                                n2023 = call "waveformsDObuffer.vi"("DO wf in"=w5190, "command"="set") -> ()  [unwired: 1 out]
                                }
                                frame True {
                                }
                                }
                                }
                                }
                                }
                                }
                                }
                                }
                              }
                              frame #3 {
                                n2024 = Build Array(w5197, w5196) -> (w5198:bool[])
                                n2025 = Boolean Array To Number(Boolean array=w5198) -> (number=w5195:u32)
                                n2026 = case shown="0" w5195 {
                                tunnel: w5202 -> [_ _ w5245]
                                tunnel: w5201 -> [_ _ w5244]
                                tunnel: w5200 -> [_ w5224 w5242]
                                tunnel: w5199 -> [_ w5223 w5243]
                                frame 1, Default {
                                n2027 = stacked-sequence {
                                seq-local: [w5205 _ _] -> [_ w5215 w5220]
                                frame #0 {
                                n2028 = call "configuration_2P_Linlin.vi"("command"="get") -> ("config out"=w5203:T14)  [unwired: 2 in, 1 out]
                                n2029 = Unbundle By Name(w5203) -> ("LT timestamp"=w5208:u32)
                                n2030 = call "2pparameters.vi"("command"="get") -> ("params out"=w5209:T12)  [unwired: 1 in]
                                n2031 = in-place {
                                in-place-border: w5208 -> [w5214]
                                in-place-border: [w5211] -> w5205
                                n2032 = in-place-cluster #41(w5209) -> ("aDO"=w5213:u32[])
                                n2033 = call "remove channel from active arrayv2.vi"("line array in"=w5213, "line to remove"=w5214) -> ("line array out"=w5212:u32[], "index"=w5211:i32)  [unwired: 1 out]
                                n2034 = in-place-cluster #41("aDO"=w5212) -> (w5206:T12)
                                }
                                n2035 = call "2pparameters.vi"("Params in"=w5206, "command"="set") -> ()  [unwired: 1 out]
                                }
                                frame #1 {
                                n2036 = call "waveformparamsv2.vi"("command"="rem DO", "index"=w5215) -> ()  [unwired: 3 in, 3 out]
                                }
                                frame #2 {
                                n2037 = call "waveformsDObuffer.vi"("command"="get") -> ("DO wf out"=w5221:digitalwaveform[])  [unwired: 1 in]
                                n2038 = Delete From Array(array=w5221, length=1, index=w5220) -> (array with subset deleted=w5217:digitalwaveform[])  [unwired: 1 out]
                                n2039 = call "waveformsDObuffer.vi"("DO wf in"=w5217, "command"="set") -> ()  [unwired: 1 out]
                                }
                                }
                                }
                                frame 2 {
                                n2040 = stacked-sequence {
                                tunnel: w5224 -> [_ _ w5237]
                                tunnel: w5223 -> [_ w5235 _]
                                frame #0 {
                                n2041 = call "configuration_2P_Linlin.vi"("command"="get") -> ("config out"=w5225:T14)  [unwired: 2 in, 1 out]
                                n2042 = Unbundle By Name(w5225) -> ("LT timestamp"=w5227:u32)
                                n2043 = call "2pparameters.vi"("command"="get") -> ("params out"=w5230:T12)  [unwired: 1 in]
                                n2044 = in-place {
                                in-place-border: w5227 -> [w5234]
                                n2045 = in-place-cluster #42(w5230) -> ("aDO"=w5233:u32[])
                                n2046 = call "add channel to active arrayv2.vi"("line array in"=w5233, "line to add"=w5234) -> ("line array out"=w5232:u32[])  [unwired: 2 out]
                                n2047 = in-place-cluster #42("aDO"=w5232) -> (w5228:T12)
                                }
                                n2048 = call "2pparameters.vi"("Params in"=w5228, "command"="set") -> ()  [unwired: 1 out]
                                }
                                frame #1 {
